vi "Dealt Cards String to Card Map Indices.vi"(11 "Dealt Cards String":string) -> (2 "Index1":i32, 3 "Index0":i32)   [LabVIEW 2021]
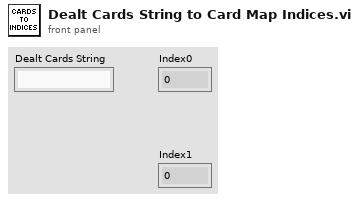
[diagram p1: front panel]
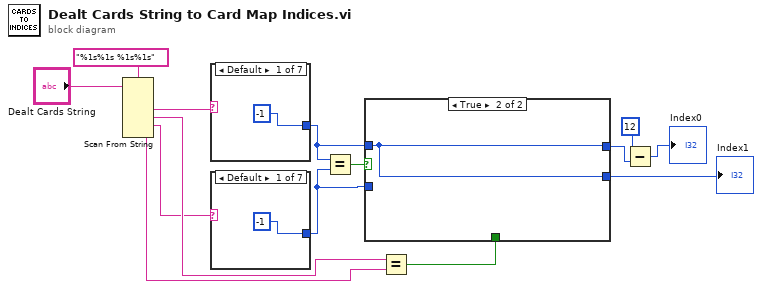
[diagram p0: block diagram]
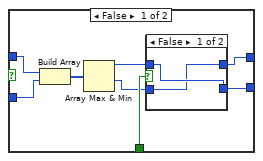
[diagram p2: hidden frame]
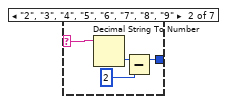
[diagram p4: hidden frame]
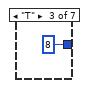
[diagram p5: hidden frame]
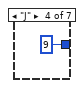
[diagram p6: hidden frame]
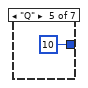
[diagram p7: hidden frame]
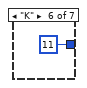
[diagram p8: hidden frame]
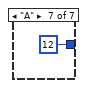
[diagram p9: hidden frame]
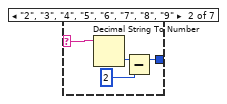
[diagram p10: hidden frame]
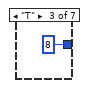
[diagram p11: hidden frame]
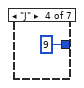
[diagram p12: hidden frame]
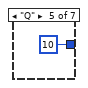
[diagram p13: hidden frame]
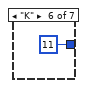
[diagram p14: hidden frame]
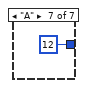
[diagram p15: hidden frame]
diagram:
  n1 = Scan From String(format string="%1s%1s %1s%1s", input string="Dealt Cards String") -> (output 1=w3:string, output 2=w8:string, output 3=w4:string, output 4=w9:string)  [unwired: 6 in, 3 out]
  n2 = case shown="Default" w3 {
    selector: w3 -> [_ w19 _ _ _ _ _]
    tunnel: [-1 w17 8 9 10 11 12] -> w6
    frame Default {
    }
    frame "2", "3", "4", "5", "6", "7", "8", "9" {
      n3 = Decimal String To Number(string=w19) -> (number=w18:i32)  [unwired: 2 in, 1 out]
      n4 = Subtract(x=w18, y=2) -> (x-y=w17:i32)
    }
    frame "T" {
    }
    frame "J" {
    }
    frame "Q" {
    }
    frame "K" {
    }
    frame "A" {
    }
  }
  n5 = case shown="Default" w4 {
    selector: w4 -> [_ w29 _ _ _ _ _]
    tunnel: [-1 w27 8 9 10 11 12] -> w7
    frame Default {
    }
    frame "2", "3", "4", "5", "6", "7", "8", "9" {
      n6 = Decimal String To Number(string=w29) -> (number=w28:i32)  [unwired: 2 in, 1 out]
      n7 = Subtract(x=w28, y=2) -> (x-y=w27:i32)
    }
    frame "T" {
    }
    frame "J" {
    }
    frame "Q" {
    }
    frame "K" {
    }
    frame "A" {
    }
  }
  n8 = Equal?(x=w6, y=w7) -> (x = y?=w5:bool)
  n9 = Equal?(x=w8, y=w9) -> (x = y?=w10:bool)
  n10 = case shown="True" w5 {
    tunnel: [w36 w47] -> w13
    tunnel: w6 -> [w42 w47]
    tunnel: [w35 w47] -> w11
    tunnel: w7 -> [w41 _]
    tunnel: w10 -> [w39 _]
    frame False {
      n11 = Build Array(w42, w41) -> (w40:i32[])
      n12 = Array Max & Min(array=w40) -> (max value=w37:i32, min value=w38:i32)  [unwired: 2 out]
      n13 = case shown="False" w39 {
        tunnel: w38 -> [w43 w45]
        tunnel: w37 -> [w44 w46]
        tunnel: [w43 w46] -> w36
        tunnel: [w44 w45] -> w35
        frame False {
        }
        frame True {
        }
      }
    }
    frame True {
    }
  }
  "Index1" <- w11
  n14 = Subtract(x=12, y=w13) -> (x-y=→"Index0":i32)
